vi "string_begins_with.vi"(1 "String to compare":string, 2 "Beginning string":string) -> (0 "Begins with?":bool)   [LabVIEW 2015]
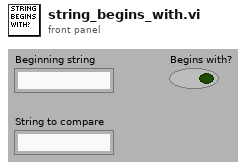
[diagram p1: front panel]
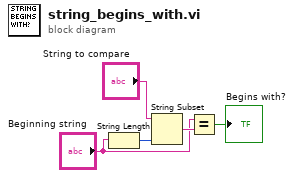
[diagram p0: block diagram]
diagram:
  n1 = String Length(string="Beginning string") -> (length=w1:i32)
  n2 = String Subset(string="String to compare", length (rest)=w1) -> (substring=w5:string)  [unwired: 1 in]
  n3 = Equal?(x="Beginning string", y=w5) -> (x = y?=→"Begins with?":bool)
